vi "Get G Score.vi"(10 "Position":cluster{"Row":i32, "Col":i32}, 11 "Map":T1) -> (2 "gScore":i32)   [LabVIEW 2022 SP3, in "AoC22.lvlib"]
uses:
  AoC22.lvlib
  Map.ctl
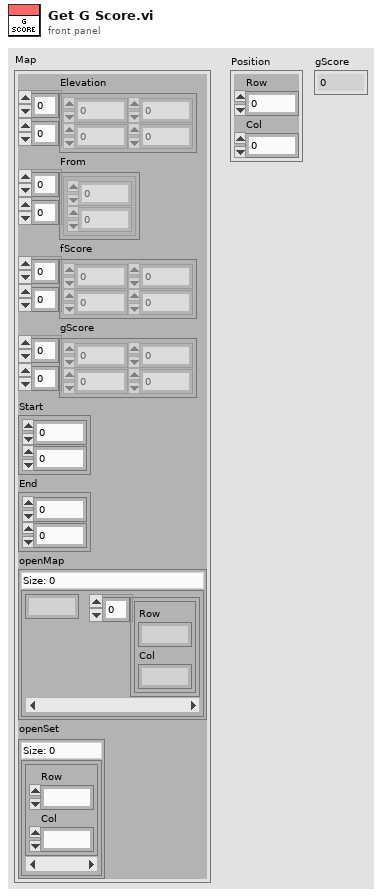
[diagram p1: front panel]
types:
  T1 = typedef "AoC22.lvlib/Map.ctl" = cluster{"Elevation":u8[][], "From":cluster{"Row":i32, "Col":i32}[][], "fScore":i32[][], "gScore":i32[][], "Start":cluster{"Row":i32, "Col":i32}, "End":cluster{"Row":i32, "Col":i32}, "openMap":map{i32, cluster{"Row":i32, "Col":i32}[]}, "openSet":set{cluster{"Row":i32, "Col":i32}}}
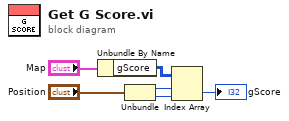
[diagram p0: block diagram]
diagram:
  n1 = Unbundle By Name("Map") -> ("gScore"=w5:i32[][])
  n2 = Unbundle("Position") -> ("Row"=w3:i32, "Col"=w2:i32)
  n3 = Index Array(array=w5, index (row)=w3, index (col)=w2) -> (element=→"gScore":i32)
